vi "Actor Core.vi"(8 "error in":errorcluster, 11 "LTI ULS Actor in":refnum<class "LTI ULS Actor.lvclass">) -> (0 "error out":errorcluster, 3 "LTI ULS Actor out":refnum<class "Actor.lvclass">)   [LabVIEW 2018, in "LTI ULS Actor.lvlib" / "LTI ULS Actor.lvclass"]
doc: "(<B>Filename</B>: Actor Framework.lvlib:Actor.lvclass:Actor Core.vi)\n\nReceives messages to the actor, reacts to them, and initiates any error handling that may shut the actor down.\n\nDescendant classes may override this VI to append parallel tasks for the actor to complete while it handles messages. Overrides use the Call Parent Method node."
uses:
  LTI ULS Actor.lvclass
  C:/Program Files (x86)/National Instruments/LabVIEW 2018/vi.lib/ActorFramework/Actor/Actor.lvclass
  <vilib>/ActorFramework/Actor/Actor.lvclass
  <vilib>/ActorFramework/Actor/Actor.lvclass/Actor.ctl
  <vilib>/ActorFramework/Message Enqueuer/Message Enqueuer.lvclass/Message Enqueuer.ctl
  LTI ULS Actor.lvclass/LTI ULS Actor.ctl
  <vilib>/ActorFramework/Message Enqueuer/Init from Existing Queue.vi
  <vilib>/ActorFramework/Message Enqueuer/Enqueue.vi
  <vilib>/ActorFramework/Stop Msg/Stop Msg.lvclass
  C:/Program Files (x86)/National Instruments/LabVIEW 2018/vi.lib/ActorFramework/Message/Message.lvclass
  <vilib>/ActorFramework/Message Priority Queue/Priority Enqueue.vi
  Sensor Actor/Sensor/Sensor.lvclass
  <vilib>/ActorFramework/Message Enqueuer/Message Enqueuer.lvclass
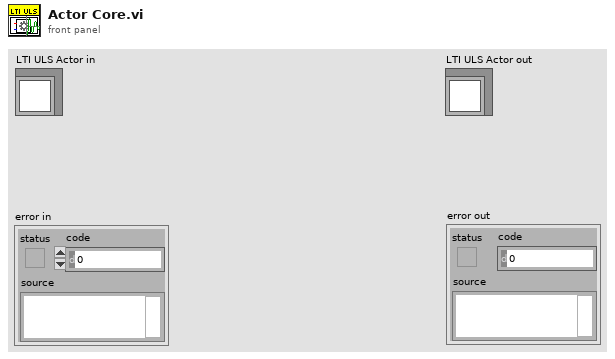
[diagram p1: front panel]
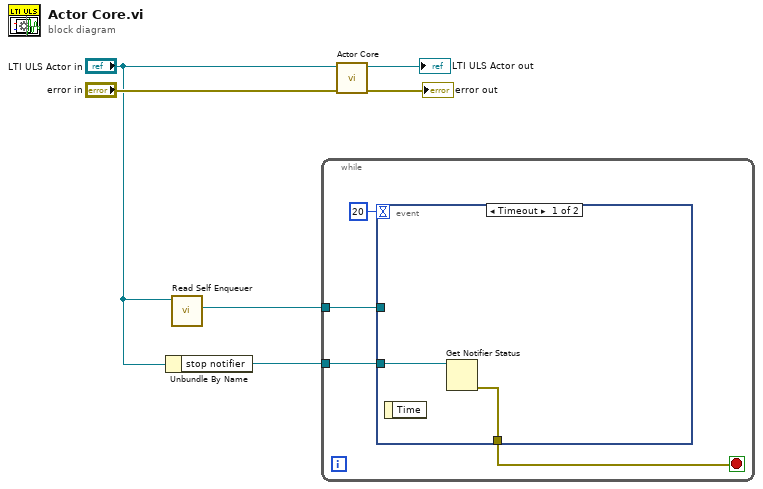
[diagram p0: block diagram]
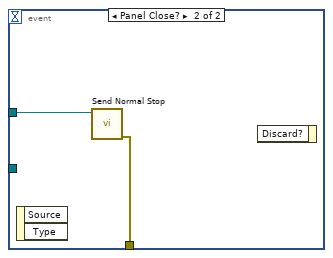
[diagram p2: hidden frame]
diagram:
  n1 = Unbundle By Name("LTI ULS Actor in") -> ("stop notifier"=w1:refnum<notifier>)
  n2 = call <vilib>:"Read Self Enqueuer.vi"("Actor"="LTI ULS Actor in") -> ("Self Enqueuer"=w2:refnum<class "Message Enqueuer.lvclass">)  [unwired: 10 in]
  n3 = while {
    tunnel: w2 -> [w8]
    tunnel: w1 -> [w7]
    stop <- w9 stop-if-true
    n4 = event shown="[0] Timeout" {
      selector: _ -> [_ _]
      dyn-events: _ -> [_ _]
      timeout: 20 -> [_ _]
      tunnel: [w12 w14] -> w9
      tunnel: w8 -> [_ w13]
      tunnel: w7 -> [w11 _]
      event Timeout {
        n5 = event-data() -> ()  [unwired: 1 in, 1 out]
        n6 = Get Notifier Status(notifier=w11) -> (error out=w12:errorcluster)  [unwired: 1 in, 4 out]
      }
      event Panel Close? {
        n7 = event-data() -> ()  [unwired: 1 in, 2 out]
        n8 = call <vilib>:"Send Normal Stop.vi"("Message Enqueuer"=w13) -> ("error out"=w14:errorcluster)  [unwired: 10 in]
        n9 = event-data() -> ()  [unwired: 2 in, 1 out]
      }
    }
  }
  n10 = call-parent "Actor Core.vi"("error in"="error in", "Sensor in"="LTI ULS Actor in") -> ("error out"=→"error out":errorcluster, "Actor out"=→"LTI ULS Actor out":refnum<class "Actor.lvclass">)  [unwired: 8 in]
